vi "ConditionallySerialiaze.vi"(8 "error in (no error)":errorcluster, 11 "Device Item Ref in":T1 format="%.0x") -> (0 "error out":errorcluster)   [LabVIEW 2016, in "Ballard Arinc-429 System Explorer.lvlib"]
uses:
  Ballard Arinc-429 System Explorer.lvlib
  <vilib>/NI Veristand/Custom Device API/Custom Device Item Ref.ctl
  <vilib>/NI Veristand/Custom Device API/Custom Device API.lvlib
  Shared/Controls and Global/Global.vi
  Shared/Ballard Arinc-429 Shared.lvlib
  <vilib>/NI Veristand/Custom Device API/Get Item Property (Path).vi
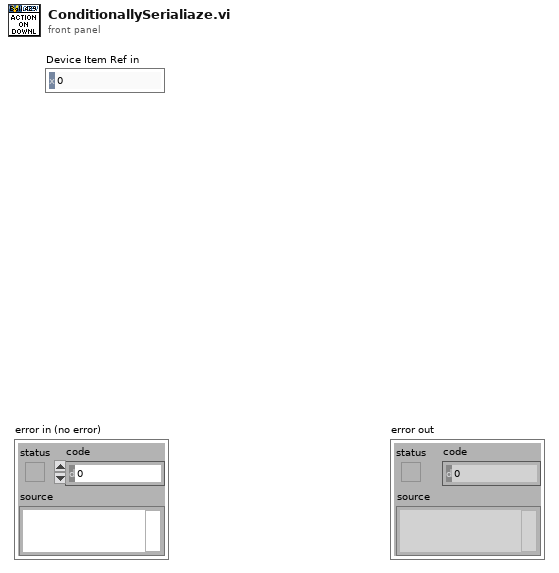
[diagram p1: front panel]
types:
  T1 = typedef "Custom Device API.lvlib/Custom Device Item Ref.ctl" = u64
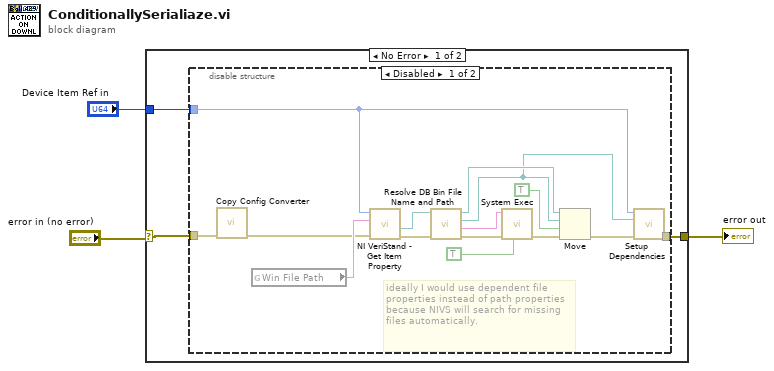
[diagram p0: block diagram]
diagram:
  n1 = case shown="No Error" "error in (no error)" {
    selector: "error in (no error)" -> [w4 w22]
    tunnel: [w6 w22] -> w3
    tunnel: "Device Item Ref in" -> [w5 _]
    frame No Error {
      n2 = disable-structure shown="Disabled" {
        disable-tunnel: [w20 _] -> w6
        disable-tunnel: w5 -> [w19 _]
        disable-tunnel: w4 -> [w8 _]
        frame Disabled {
          # "ideally I would use dependent file properties instead of path properties because NIVS will search for missing files automatically."
          n3 = call "Copy Config Converter.vi"("error in (no error)"=w8) -> ("error out"=w7:errorcluster)  [unwired: 10 in]
          n4 = global read "Global.vi" "Win File Path"() -> (w21:string)
          n5 = call-poly <vilib>:"NI VeriStand - Get Item Property.vi"("error in (no error)"=w7, "Property Name"=w21, "Item Ref in"=w19) -> ("error out"=w16:errorcluster, "Value"=w12:path)  [unwired: 5 in, 2 out]
          n6 = call "Resolve DB Bin File Name and Path.vi"("error in"=w16, "DB XML File"=w12) -> ("error out"=w15:errorcluster, "SysExec"=w11:string, "Destination File"=w9:path, "Converted File"=w10:path)  [unwired: 6 in]
          n7 = call <vilib>:"System Exec.vi"("run minimized? (F)"=TRUE, "error in (no error)"=w15, "command line"=w11) -> ("error out"=w14:errorcluster)  [unwired: 5 in, 3 out]
          n8 = Move(source path=w10, error in=w14, 9:TRUE ("overwrite (F)"), 10:w9) -> (error out=w13:errorcluster)  [unwired: 1 in, 2 out]
          n9 = call "Setup Dependencies.vi"("error in (no error)"=w13, "Windows Bin File"=w9, "Item Ref in"=w19) -> ("error out"=w20:errorcluster)  [unwired: 8 in]
        }
        frame Enabled {
        }
      }
    }
    frame Error {
    }
  }
  "error out" <- w3
